vi "InverseMpemba_HotColdWarm.vi"(6 "RN":sgl, 8 "X0":sgl=0.5, 11 "Ring":i16(ring) items=["Cold", "Warm", "Hot"]) -> (3 "Xpot":sgl)   [LabVIEW 2019]
uses:
  <vilib>/Platform/TimedLoop/XDataNode/timing_clust.ctl
  <vilib>/Platform/TimedLoop/XDataNode/nitl_modes.ctl
  <vilib>/Platform/TimedLoop/XDataNode/wakeup.ctl
  <vilib>/rvi/Emulation/niFpgaGetClockAttributes.vi
  <vilib>/rvi/Emulation/niFpgaSctlEmulationGetInTimedLoop.vi
  <vilib>/rvi/Emulation/niFpgaEmulationReportErrorSimple.vi
  <vilib>/rvi/Emulation/niFpgaCriticalErrorInLSC.vi
  <vilib>/Platform/TimedLoop/XDataNode/XDataNode.xnode
  <vilib>/Platform/TimedLoop/XDataNode/XDNodeRunTimeDep.lvlib
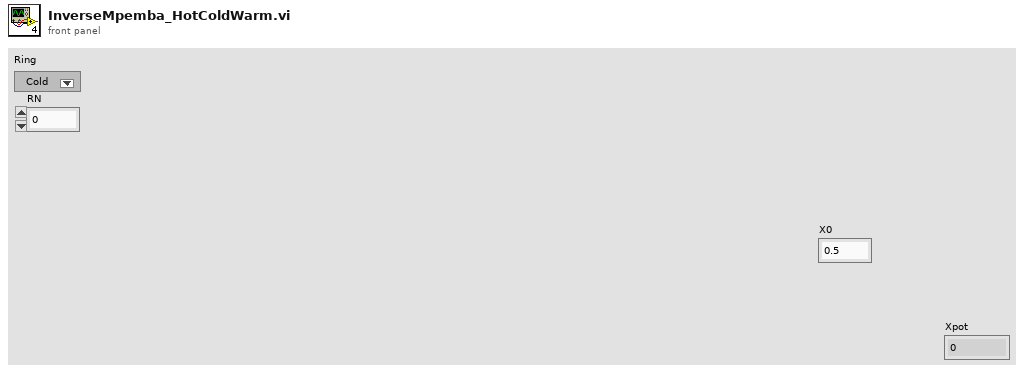
[diagram p1: front panel]
types:
  T1 = typedef "XDNodeRunTimeDep.lvlib/timing_clust.ctl" = cluster{"Expected End [f-1]":u64, "Actual End [f-1]":u64, "Finished Late? [f-1]":bool, "Expected End [i-1]":u64, "Actual End [i-1]":u64, "Finished Late? [i-1]":bool, "Expected Start [i]":u64, "Actual Start [i]":u64, "Expected Start [f]":u64, "Actual Start [f]":u64, "Source Name":string, "Structure Name":string, "Period":i64, "Deadline":i64, "Offset":i64, "Start":i64, "Priority":i32, "Timeout":i32, "Mode":T2, "Wakeup Reason":T3, "Error":errorcluster, "Source Type":string, "Secondary Source Type":string, "Global End Time":u64, "Global Start Time":u64, "Frame Duration":u64, "Iteration Duration":u64, "Assigned CPU":i32, "I/O Scan Engine Mode":u32}
  T2 = typedef "XDNodeRunTimeDep.lvlib/nitl_modes.ctl" = enum32{"No Change", "Process missed periods, maintain original phase", "Discard missed periods, maintain original phase", "Process missed periods, ignore original phase", "Discard missed periods, ignore original phase"}
  T3 = typedef "XDNodeRunTimeDep.lvlib/wakeup.ctl" = enum32{"Normal", "Aborted", "Asynchronous wakeup", "Timing source error", "Timed loop error", "Timeout"}
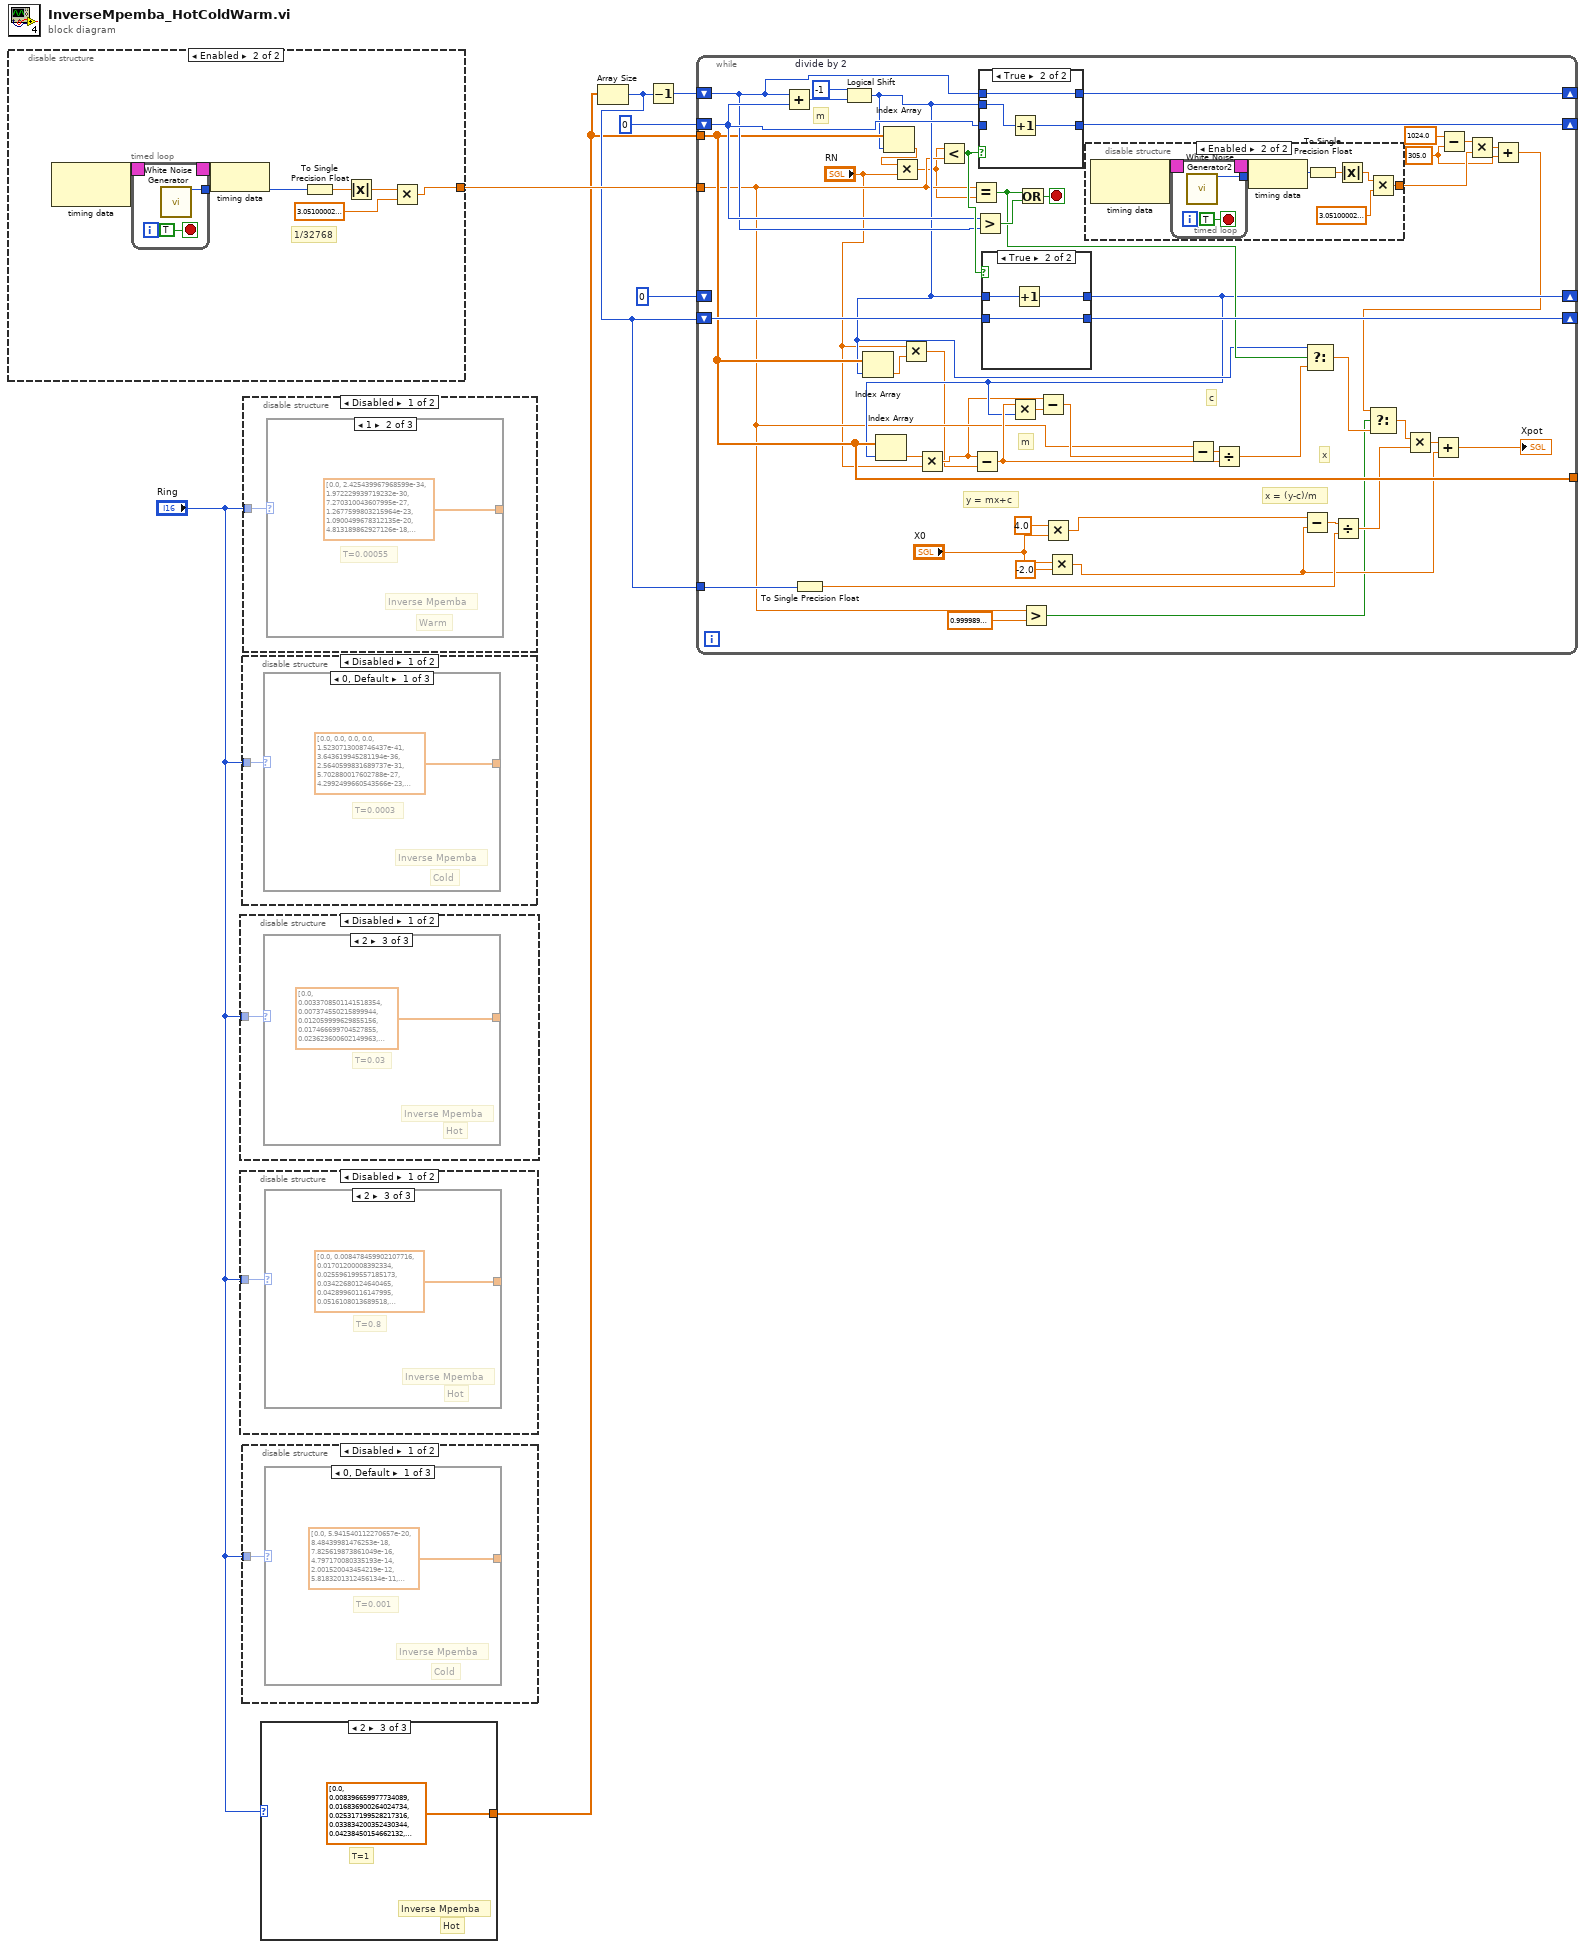
[diagram p0: block diagram]
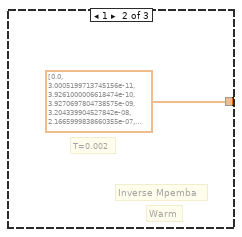
[diagram p2: hidden frame]
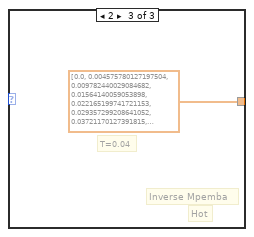
[diagram p3: hidden frame]
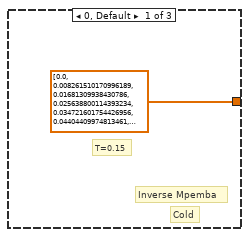
[diagram p5: hidden frame]
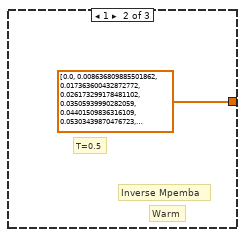
[diagram p6: hidden frame]
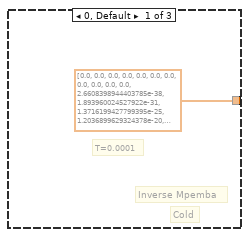
[diagram p7: hidden frame]
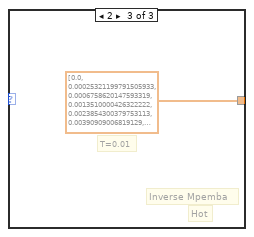
[diagram p8: hidden frame]
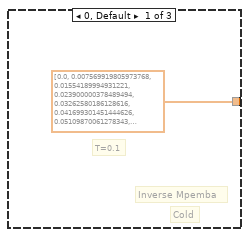
[diagram p10: hidden frame]
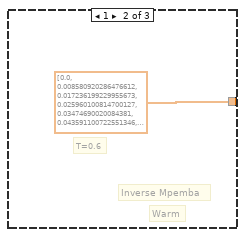
[diagram p11: hidden frame]
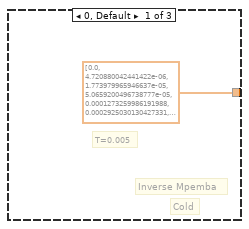
[diagram p13: hidden frame]
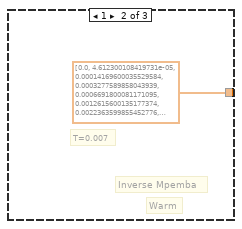
[diagram p14: hidden frame]
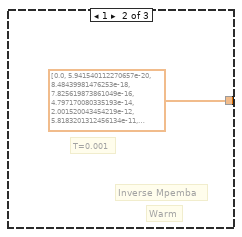
[diagram p16: hidden frame]
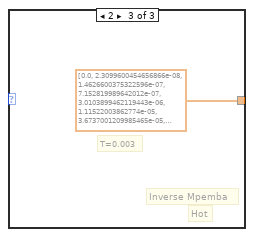
[diagram p17: hidden frame]
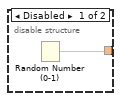
[diagram p19: hidden frame]
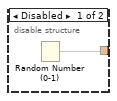
[diagram p20: hidden frame]
diagram:
  n1 = disable-structure shown="Enabled" {
    disable-tunnel: [w8 w11] -> w4
    frame Disabled {
      n2 = Random Number (0-1)() -> (number: 0 to 1=w8:dbl)
    }
    frame Enabled {
      # "1/32768"
      n3 = node-c288() -> (w10:T1)  [unwired: 1 in]
      n4 = timed-loop {
        timing: w10 -> [_]
        timing-out: [_] -> w9
        tunnel: [w17] -> w15
        stop <- TRUE stop-if-true
        n5 = call "White Noise Generator"() -> ("white noise out"=w17:i16)  [unwired: 15 in]
      }
      n6 = node-c288(w9) -> ()
      n7 = To Single Precision Float(number=w15) -> (single precision float=w13:sgl)
      n8 = Absolute Value(x=w13) -> (abs(x)=w12:sgl)
      n9 = Multiply(x=w12, y=sgl 3.051e-05) -> (x*y=w11:sgl)
    }
  }
  n10 = disable-structure shown="Disabled" {
    disable-tunnel: "Ring" -> [w22 _]
    frame Disabled {
      n11 = case shown="2" w22 {
        tunnel: [sgl[] [0.0, 4.72088e-06, 1.77398e-05, 5.06592e-05, 0.000127326, 0.000292503, 0.000623122, 0.0012405, 0.0023204, 0.00409678, 0.00685531, 0.0109145, 0.016595, 0.024182, 0.0338863, 0.0458131, 0.0599432, 0.0761305, 0.0941165, 0.113555, 0.134049, 0.15518, 0.176546, 0.197782, 0.218581, 0.238699, 0.257958, 0.276241, 0.293487, 0.309682, 0.324844, 0.339022, 0.352281, 0.364701, 0.376365, 0.387364, 0.397785, 0.407716, 0.417243, 0.426449, 0.435413, 0.444214, 0.452928, 0.461633, 0.470404, 0.47932, 0.488461, 0.497912, 0.50776, 0.518098, 0.529026, 0.540646, 0.553068, 0.566402, 0.580761, 0.596254, 0.612981, 0.631025, 0.650444, 0.67126, 0.693445, 0.716907, 0.741482, 0.766922, 0.79289, 0.81897, 0.844674, 0.869473, 0.892834, 0.914258, 0.933335, 0.949775, 0.963448, 0.974386, 0.982774, 0.988922, 0.993211, 0.996051, 0.997828, 0.998875, 0.999453, 0.999752, 0.999895, 0.999959, 0.999985, 0.999995, 0.999999, 1.0, 1.0, 1.0, 1.0, 1.0, 1.0, 1.0, 1.0, 1.0, 1.0, 1.0, 1.0, 1.0, 1.0, 1.0, 1.0, 1.0, 1.0, 1.0, 1.0, 1.0, 1.0, 1.0, 1.0, 1.0, 1.0, 1.0, 1.0, 1.0, 1.0, 1.0, 1.0, 1.0, 1.0, 1.0, 1.0, 1.0, 1.0, 1.0, 1.0, 1.0] ("Init Data Out") sgl[] [0.0, 4.6123e-05, 0.000141696, 0.000327759, 0.00066918, 0.00126156, 0.00223636, 0.00376235, 0.0060415, 0.00929849, 0.0137642, 0.0196549, 0.02715, 0.0363724, 0.0473733, 0.0601252, 0.074523, 0.0903924, 0.107505, 0.125596, 0.144383, 0.163587, 0.182944, 0.202216, 0.221204, 0.239745, 0.257717, 0.275033, 0.291642, 0.30752, 0.322669, 0.337109, 0.350874, 0.36401, 0.376572, 0.388616, 0.400206, 0.411404, 0.422275, 0.432883, 0.443291, 0.453564, 0.463765, 0.473957, 0.484205, 0.494573, 0.505128, 0.515936, 0.527067, 0.538591, 0.550581, 0.563108, 0.576246, 0.590066, 0.604637, 0.62002, 0.636269, 0.653422, 0.671499, 0.690496, 0.710378, 0.731071, 0.752462, 0.774387, 0.796638, 0.818956, 0.841044, 0.862574, 0.883202, 0.902591, 0.920434, 0.936475, 0.950531, 0.962511, 0.972417, 0.980344, 0.986469, 0.991025, 0.99428, 0.996507, 0.997962, 0.998868, 0.999403, 0.999702, 0.999859, 0.999938, 0.999974, 0.99999, 0.999996, 0.999999, 1.0, 1.0, 1.0, 1.0, 1.0, 1.0, 1.0, 1.0, 1.0, 1.0, 1.0, 1.0, 1.0, 1.0, 1.0, 1.0, 1.0, 1.0, 1.0, 1.0, 1.0, 1.0, 1.0, 1.0, 1.0, 1.0, 1.0, 1.0, 1.0, 1.0, 1.0, 1.0, 1.0, 1.0, 1.0, 1.0, 1.0, 1.0] ("Init Data Out") sgl[] [0.0, 0.00337085, 0.00737455, 0.01206, 0.0174667, 0.0236236, 0.0305473, 0.0382417, 0.0466981, 0.0558954, 0.0658014, 0.0763735, 0.0875612, 0.0993071, 0.111549, 0.124223, 0.137263, 0.150603, 0.164182, 0.177938, 0.191817, 0.205767, 0.219742, 0.233704, 0.247617, 0.261453, 0.275188, 0.288805, 0.30229, 0.315634, 0.328832, 0.341883, 0.35479, 0.367556, 0.38019, 0.392701, 0.4051, 0.4174, 0.429616, 0.441761, 0.453853, 0.465909, 0.477944, 0.489977, 0.502026, 0.514107, 0.526239, 0.538437, 0.55072, 0.563103, 0.5756, 0.588226, 0.600993, 0.613911, 0.62699, 0.640235, 0.653651, 0.667237, 0.680991, 0.694905, 0.708968, 0.723163, 0.737468, 0.751856, 0.766294, 0.780741, 0.795154, 0.809481, 0.823665, 0.837645, 0.851355, 0.864727, 0.877691, 0.890178, 0.90212, 0.913453, 0.924119, 0.934069, 0.943262, 0.951669, 0.959275, 0.966076, 0.972084, 0.977322, 0.981826, 0.985643, 0.988829, 0.991445, 0.993557, 0.995233, 0.996537, 0.997532, 0.998277, 0.998822, 0.999212, 0.999485, 0.999672, 0.999796, 0.999876, 0.999927, 0.999958, 0.999977, 0.999987, 0.999993, 0.999997, 0.999998, 0.999999, 1.0, 1.0, 1.0, 1.0, 1.0, 1.0, 1.0, 1.0, 1.0, 1.0, 1.0, 1.0, 1.0, 1.0, 1.0, 1.0, 1.0, 1.0, 1.0, 1.0, 1.0] ("Init Data Out")] -> _
        frame 0, Default {
          # "T=0.005"
          # "Inverse Mpemba"
          # "Cold"
        }
        frame 1 {
          # "T=0.007"
          # "Inverse Mpemba"
          # "Warm"
        }
        frame 2 {
          # "T=0.03"
          # "Inverse Mpemba"
          # "Hot"
        }
      }
    }
    frame Enabled {
    }
  }
  n12 = disable-structure shown="Disabled" {
    disable-tunnel: "Ring" -> [w26 _]
    frame Disabled {
      n13 = case shown="2" w26 {
        tunnel: [sgl[] [0.0, 0.00756992, 0.0155419, 0.0239, 0.0326258, 0.0416993, 0.0510987, 0.060801, 0.0707827, 0.0810196, 0.0914873, 0.102162, 0.113019, 0.124037, 0.135192, 0.146464, 0.157833, 0.16928, 0.180787, 0.19234, 0.203924, 0.215525, 0.227133, 0.238737, 0.25033, 0.261903, 0.27345, 0.284968, 0.296452, 0.307899, 0.31931, 0.330682, 0.342016, 0.353313, 0.364574, 0.375803, 0.387001, 0.398173, 0.409321, 0.42045, 0.431565, 0.442669, 0.453768, 0.464866, 0.475968, 0.48708, 0.498205, 0.509349, 0.520516, 0.53171, 0.542935, 0.554194, 0.565491, 0.576828, 0.588207, 0.59963, 0.611096, 0.622606, 0.634158, 0.64575, 0.65738, 0.669042, 0.680731, 0.692441, 0.704162, 0.715887, 0.727602, 0.739297, 0.750956, 0.762565, 0.774106, 0.785561, 0.79691, 0.808131, 0.819203, 0.830103, 0.840806, 0.851287, 0.861522, 0.871486, 0.881155, 0.890504, 0.89951, 0.908153, 0.916412, 0.92427, 0.931712, 0.938726, 0.945303, 0.951436, 0.957124, 0.962368, 0.967173, 0.971547, 0.975503, 0.979054, 0.98222, 0.98502, 0.987478, 0.989617, 0.991463, 0.993042, 0.99438, 0.995504, 0.996437, 0.997206, 0.997831, 0.998334, 0.998735, 0.999051, 0.999296, 0.999484, 0.999627, 0.999734, 0.999813, 0.99987, 0.999911, 0.99994, 0.99996, 0.999974, 0.999984, 0.99999, 0.999994, 0.999996, 0.999998, 0.999999, 1.0, 1.0] ("Init Data Out") sgl[] [0.0, 0.00858092, 0.0172362, 0.0259601, 0.0347469, 0.0435911, 0.0524875, 0.0614311, 0.0704172, 0.0794412, 0.0884988, 0.097586, 0.106699, 0.115834, 0.124988, 0.134158, 0.143342, 0.152535, 0.161737, 0.170945, 0.180157, 0.189371, 0.198586, 0.207801, 0.217014, 0.226224, 0.235431, 0.244634, 0.253833, 0.263027, 0.272215, 0.281399, 0.290578, 0.299751, 0.30892, 0.318084, 0.327244, 0.3364, 0.345554, 0.354704, 0.363853, 0.373, 0.382147, 0.391293, 0.40044, 0.409588, 0.418738, 0.427891, 0.437047, 0.446206, 0.45537, 0.464538, 0.473712, 0.482891, 0.492075, 0.501266, 0.510462, 0.519664, 0.528872, 0.538085, 0.547303, 0.556525, 0.565751, 0.574979, 0.584209, 0.59344, 0.602669, 0.611895, 0.621117, 0.630333, 0.639539, 0.648734, 0.657914, 0.667077, 0.67622, 0.685339, 0.69443, 0.70349, 0.712513, 0.721497, 0.730435, 0.739323, 0.748157, 0.756929, 0.765636, 0.774271, 0.782827, 0.7913, 0.799681, 0.807966, 0.816148, 0.824219, 0.832173, 0.840003, 0.847703, 0.855266, 0.862685, 0.869954, 0.877066, 0.884015, 0.890795, 0.8974, 0.903826, 0.910066, 0.916117, 0.921974, 0.927632, 0.93309, 0.938344, 0.943391, 0.948231, 0.952861, 0.957282, 0.961494, 0.965497, 0.969293, 0.972884, 0.976272, 0.979461, 0.982455, 0.985258, 0.987875, 0.990311, 0.992573, 0.994665, 0.996596, 0.998372, 1.0] ("Init Data Out") sgl[] [0.0, 0.00847846, 0.017012, 0.0255962, 0.0342268, 0.0428996, 0.0516108, 0.0603567, 0.0691336, 0.0779384, 0.0867677, 0.0956186, 0.104488, 0.113374, 0.122274, 0.131186, 0.140107, 0.149035, 0.15797, 0.166909, 0.175851, 0.184794, 0.193738, 0.202682, 0.211625, 0.220566, 0.229504, 0.23844, 0.247372, 0.256301, 0.265226, 0.274147, 0.283064, 0.291978, 0.300889, 0.309796, 0.3187, 0.327602, 0.336501, 0.345398, 0.354294, 0.363189, 0.372083, 0.380977, 0.389871, 0.398767, 0.407664, 0.416563, 0.425464, 0.434367, 0.443274, 0.452184, 0.461098, 0.470016, 0.478938, 0.487864, 0.496795, 0.505729, 0.514668, 0.523611, 0.532557, 0.541507, 0.550459, 0.559413, 0.568368, 0.577323, 0.586278, 0.59523, 0.604179, 0.613124, 0.622062, 0.630991, 0.63991, 0.648816, 0.657708, 0.666582, 0.675436, 0.684267, 0.693071, 0.701846, 0.710588, 0.719293, 0.727958, 0.736578, 0.74515, 0.753668, 0.762128, 0.770526, 0.778857, 0.787115, 0.795295, 0.803393, 0.811403, 0.819319, 0.827136, 0.834848, 0.84245, 0.849936, 0.8573, 0.864538, 0.871644, 0.878611, 0.885436, 0.892113, 0.898637, 0.905003, 0.911208, 0.917246, 0.923114, 0.928808, 0.934326, 0.939664, 0.94482, 0.949791, 0.954577, 0.959175, 0.963586, 0.967809, 0.971845, 0.975693, 0.979356, 0.982835, 0.986133, 0.989251, 0.992193, 0.994962, 0.997563, 1.0] ("Init Data Out")] -> _
        frame 0, Default {
          # "T=0.1"
          # "Inverse Mpemba"
          # "Cold"
        }
        frame 1 {
          # "T=0.6"
          # "Inverse Mpemba"
          # "Warm"
        }
        frame 2 {
          # "T=0.8"
          # "Inverse Mpemba"
          # "Hot"
        }
      }
    }
    frame Enabled {
    }
  }
  n14 = disable-structure shown="Disabled" {
    disable-tunnel: "Ring" -> [w30 _]
    frame Disabled {
      n15 = case shown="0, Default" w30 {
        tunnel: [sgl[] [0.0, 0.0, 0.0, 0.0, 1.52307e-41, 3.64362e-36, 2.56406e-31, 5.70288e-27, 4.29925e-23, 1.17597e-19, 1.2472e-16, 5.4725e-14, 1.05882e-11, 9.62107e-10, 4.37214e-08, 1.05841e-06, 1.45426e-05, 0.000120786, 0.000644813, 0.00234578, 0.00614557, 0.0122228, 0.0194327, 0.025991, 0.0307127, 0.0334893, 0.034865, 0.0354572, 0.0356854, 0.0357664, 0.0357937, 0.0358026, 0.0358055, 0.0358065, 0.0358068, 0.035807, 0.035807, 0.035807, 0.0358071, 0.0358071, 0.0358071, 0.0358071, 0.0358071, 0.0358071, 0.0358071, 0.0358071, 0.0358071, 0.0358071, 0.0358071, 0.0358072, 0.0358073, 0.0358076, 0.0358086, 0.0358119, 0.0358233, 0.0358639, 0.0360097, 0.0365221, 0.0382423, 0.0436096, 0.0587325, 0.0960808, 0.174483, 0.310085, 0.49734, 0.69738, 0.857477, 0.950293, 0.987861, 0.998043, 0.999804, 0.999989, 1.0, 1.0, 1.0, 1.0, 1.0, 1.0, 1.0, 1.0, 1.0, 1.0, 1.0, 1.0, 1.0, 1.0, 1.0, 1.0, 1.0, 1.0, 1.0, 1.0, 1.0, 1.0, 1.0, 1.0, 1.0, 1.0, 1.0, 1.0, 1.0, 1.0, 1.0, 1.0, 1.0, 1.0, 1.0, 1.0, 1.0, 1.0, 1.0, 1.0, 1.0, 1.0, 1.0, 1.0, 1.0, 1.0, 1.0, 1.0, 1.0, 1.0, 1.0, 1.0, 1.0, 1.0, 1.0, 1.0] ("Init Data Out") sgl[] [0.0, 5.94154e-20, 8.4844e-18, 7.82562e-16, 4.79717e-14, 2.00152e-12, 5.81832e-11, 1.20575e-09, 1.82176e-08, 2.05116e-07, 1.75793e-06, 1.17058e-05, 6.1769e-05, 0.000263223, 0.000922445, 0.00270504, 0.00674966, 0.0145632, 0.0275964, 0.0466214, 0.0712428, 0.0998487, 0.130049, 0.159361, 0.185814, 0.208252, 0.226325, 0.240289, 0.250735, 0.258369, 0.263866, 0.267796, 0.270606, 0.272631, 0.27411, 0.27521, 0.276049, 0.276708, 0.277242, 0.277691, 0.278084, 0.278443, 0.278784, 0.279123, 0.279475, 0.279857, 0.280291, 0.280804, 0.281436, 0.282242, 0.283308, 0.28476, 0.28679, 0.289687, 0.293886, 0.300029, 0.30904, 0.322196, 0.34117, 0.367978, 0.404757, 0.453305, 0.514361, 0.586776, 0.666913, 0.748743, 0.82496, 0.888943, 0.936757, 0.96816, 0.986048, 0.994764, 0.998345, 0.999567, 0.999908, 0.999984, 0.999998, 1.0, 1.0, 1.0, 1.0, 1.0, 1.0, 1.0, 1.0, 1.0, 1.0, 1.0, 1.0, 1.0, 1.0, 1.0, 1.0, 1.0, 1.0, 1.0, 1.0, 1.0, 1.0, 1.0, 1.0, 1.0, 1.0, 1.0, 1.0, 1.0, 1.0, 1.0, 1.0, 1.0, 1.0, 1.0, 1.0, 1.0, 1.0, 1.0, 1.0, 1.0, 1.0, 1.0, 1.0, 1.0, 1.0, 1.0, 1.0, 1.0, 1.0, 1.0] ("Init Data Out") sgl[] [0.0, 2.30996e-08, 1.46266e-07, 7.15282e-07, 3.01039e-06, 1.11522e-05, 3.6737e-05, 0.000108448, 0.000288933, 0.000699502, 0.00154899, 0.00315746, 0.00596125, 0.0104867, 0.0172879, 0.0268576, 0.0395304, 0.055406, 0.0743127, 0.0958207, 0.1193, 0.144005, 0.169167, 0.194078, 0.218141, 0.240907, 0.262077, 0.281493, 0.299111, 0.314975, 0.329191, 0.341902, 0.353271, 0.363464, 0.372645, 0.380968, 0.388576, 0.395596, 0.402146, 0.408332, 0.414249, 0.419987, 0.425632, 0.431265, 0.436971, 0.442835, 0.448949, 0.455411, 0.462334, 0.469841, 0.478075, 0.487199, 0.497396, 0.508873, 0.521858, 0.536597, 0.553344, 0.572345, 0.59382, 0.617927, 0.644731, 0.674153, 0.705933, 0.739594, 0.774426, 0.809506, 0.84375, 0.876018, 0.905238, 0.930553, 0.951434, 0.967756, 0.979783, 0.988095, 0.993454, 0.996658, 0.998426, 0.99932, 0.999733, 0.999905, 0.99997, 0.999991, 0.999998, 1.0, 1.0, 1.0, 1.0, 1.0, 1.0, 1.0, 1.0, 1.0, 1.0, 1.0, 1.0, 1.0, 1.0, 1.0, 1.0, 1.0, 1.0, 1.0, 1.0, 1.0, 1.0, 1.0, 1.0, 1.0, 1.0, 1.0, 1.0, 1.0, 1.0, 1.0, 1.0, 1.0, 1.0, 1.0, 1.0, 1.0, 1.0, 1.0, 1.0, 1.0, 1.0, 1.0, 1.0, 1.0] ("Init Data Out")] -> _
        frame 0, Default {
          # "T=0.0003"
          # "Inverse Mpemba"
          # "Cold"
        }
        frame 1 {
          # "T=0.001"
          # "Inverse Mpemba"
          # "Warm"
        }
        frame 2 {
          # "T=0.003"
          # "Inverse Mpemba"
          # "Hot"
        }
      }
    }
    frame Enabled {
    }
  }
  n16 = disable-structure shown="Disabled" {
    disable-tunnel: "Ring" -> [w34 _]
    frame Disabled {
      n17 = case shown="0, Default" w34 {
        tunnel: [sgl[] [0.0, 5.94154e-20, 8.4844e-18, 7.82562e-16, 4.79717e-14, 2.00152e-12, 5.81832e-11, 1.20575e-09, 1.82176e-08, 2.05116e-07, 1.75793e-06, 1.17058e-05, 6.1769e-05, 0.000263223, 0.000922445, 0.00270504, 0.00674966, 0.0145632, 0.0275964, 0.0466214, 0.0712428, 0.0998487, 0.130049, 0.159361, 0.185814, 0.208252, 0.226325, 0.240289, 0.250735, 0.258369, 0.263866, 0.267796, 0.270606, 0.272631, 0.27411, 0.27521, 0.276049, 0.276708, 0.277242, 0.277691, 0.278084, 0.278443, 0.278784, 0.279123, 0.279475, 0.279857, 0.280291, 0.280804, 0.281436, 0.282242, 0.283308, 0.28476, 0.28679, 0.289687, 0.293886, 0.300029, 0.30904, 0.322196, 0.34117, 0.367978, 0.404757, 0.453305, 0.514361, 0.586776, 0.666913, 0.748743, 0.82496, 0.888943, 0.936757, 0.96816, 0.986048, 0.994764, 0.998345, 0.999567, 0.999908, 0.999984, 0.999998, 1.0, 1.0, 1.0, 1.0, 1.0, 1.0, 1.0, 1.0, 1.0, 1.0, 1.0, 1.0, 1.0, 1.0, 1.0, 1.0, 1.0, 1.0, 1.0, 1.0, 1.0, 1.0, 1.0, 1.0, 1.0, 1.0, 1.0, 1.0, 1.0, 1.0, 1.0, 1.0, 1.0, 1.0, 1.0, 1.0, 1.0, 1.0, 1.0, 1.0, 1.0, 1.0, 1.0, 1.0, 1.0, 1.0, 1.0, 1.0, 1.0, 1.0, 1.0] ("Init Data Out") sgl[] [0.0, 3.00052e-11, 3.9261e-10, 3.92707e-09, 3.20434e-08, 2.1666e-07, 1.22831e-06, 5.90395e-06, 2.43181e-05, 8.6726e-05, 0.000270482, 0.00074488, 0.00182828, 0.0040358, 0.00808229, 0.0148089, 0.0250284, 0.0393249, 0.0578756, 0.0803594, 0.105987, 0.133639, 0.162059, 0.190055, 0.216638, 0.241106, 0.263052, 0.282331, 0.298998, 0.313241, 0.325323, 0.335539, 0.34418, 0.351515, 0.357785, 0.363197, 0.367924, 0.372115, 0.375891, 0.379355, 0.382597, 0.385692, 0.388711, 0.391722, 0.394791, 0.397989, 0.401393, 0.405094, 0.409197, 0.413832, 0.419157, 0.425369, 0.43271, 0.441476, 0.452028, 0.464788, 0.480242, 0.498918, 0.521356, 0.548039, 0.579314, 0.615274, 0.655631, 0.699613, 0.745903, 0.792685, 0.837813, 0.879109, 0.914723, 0.943477, 0.96506, 0.980014, 0.989506, 0.994985, 0.997837, 0.999166, 0.999715, 0.999915, 0.999978, 0.999995, 0.999999, 1.0, 1.0, 1.0, 1.0, 1.0, 1.0, 1.0, 1.0, 1.0, 1.0, 1.0, 1.0, 1.0, 1.0, 1.0, 1.0, 1.0, 1.0, 1.0, 1.0, 1.0, 1.0, 1.0, 1.0, 1.0, 1.0, 1.0, 1.0, 1.0, 1.0, 1.0, 1.0, 1.0, 1.0, 1.0, 1.0, 1.0, 1.0, 1.0, 1.0, 1.0, 1.0, 1.0, 1.0, 1.0, 1.0, 1.0] ("Init Data Out") sgl[] [0.0, 0.00457578, 0.00978244, 0.0156414, 0.0221652, 0.0293573, 0.0372117, 0.0457137, 0.0548401, 0.0645603, 0.0748372, 0.0856285, 0.0968879, 0.108566, 0.120613, 0.132977, 0.145608, 0.158457, 0.171477, 0.184626, 0.197861, 0.211148, 0.224453, 0.237748, 0.251009, 0.264214, 0.277347, 0.290395, 0.303348, 0.3162, 0.328946, 0.341585, 0.354119, 0.366551, 0.378887, 0.391131, 0.403294, 0.415384, 0.427411, 0.439387, 0.451323, 0.463232, 0.475126, 0.487019, 0.498923, 0.510851, 0.522816, 0.534832, 0.546909, 0.559059, 0.571294, 0.583623, 0.596056, 0.608599, 0.621258, 0.634038, 0.646941, 0.659967, 0.673114, 0.686375, 0.699742, 0.713203, 0.726743, 0.740342, 0.753975, 0.767616, 0.781232, 0.794787, 0.808241, 0.821549, 0.834663, 0.847535, 0.860111, 0.872338, 0.884162, 0.895531, 0.906394, 0.916705, 0.926421, 0.935508, 0.943936, 0.951686, 0.958746, 0.965116, 0.970804, 0.975827, 0.980213, 0.983996, 0.987217, 0.989924, 0.992167, 0.993998, 0.995471, 0.996636, 0.997542, 0.998235, 0.998755, 0.999139, 0.999415, 0.999611, 0.999747, 0.999839, 0.9999, 0.999939, 0.999964, 0.999979, 0.999988, 0.999994, 0.999997, 0.999998, 0.999999, 1.0, 1.0, 1.0, 1.0, 1.0, 1.0, 1.0, 1.0, 1.0, 1.0, 1.0, 1.0, 1.0, 1.0, 1.0, 1.0, 1.0] ("Init Data Out")] -> _
        frame 0, Default {
          # "T=0.001"
          # "Inverse Mpemba"
          # "Cold"
        }
        frame 1 {
          # "T=0.002"
          # "Inverse Mpemba"
          # "Warm"
        }
        frame 2 {
          # "T=0.04"
          # "Inverse Mpemba"
          # "Hot"
        }
      }
    }
    frame Enabled {
    }
  }
  n18 = disable-structure shown="Disabled" {
    disable-tunnel: "Ring" -> [w38 _]
    frame Disabled {
      n19 = case shown="1" w38 {
        tunnel: [sgl[] [0.0, 0.0, 0.0, 0.0, 0.0, 0.0, 0.0, 0.0, 0.0, 0.0, 0.0, 2.66084e-38, 1.89396e-31, 1.37162e-25, 1.20369e-20, 1.51581e-16, 3.22645e-13, 1.36189e-10, 1.33848e-08, 3.64184e-07, 3.36451e-06, 1.33789e-05, 2.88128e-05, 4.0894e-05, 4.58943e-05, 4.7037e-05, 4.71912e-05, 4.72046e-05, 4.72054e-05, 4.72055e-05, 4.72055e-05, 4.72055e-05, 4.72055e-05, 4.72055e-05, 4.72055e-05, 4.72055e-05, 4.72055e-05, 4.72055e-05, 4.72055e-05, 4.72055e-05, 4.72055e-05, 4.72055e-05, 4.72055e-05, 4.72055e-05, 4.72055e-05, 4.72055e-05, 4.72055e-05, 4.72055e-05, 4.72055e-05, 4.72055e-05, 4.72055e-05, 4.72055e-05, 4.72055e-05, 4.72055e-05, 4.72055e-05, 4.72055e-05, 4.72057e-05, 4.72164e-05, 4.76069e-05, 5.88841e-05, 0.000293518, 0.00350145, 0.0298047, 0.148844, 0.428559, 0.75934, 0.948955, 0.995786, 0.999894, 0.999999, 1.0, 1.0, 1.0, 1.0, 1.0, 1.0, 1.0, 1.0, 1.0, 1.0, 1.0, 1.0, 1.0, 1.0, 1.0, 1.0, 1.0, 1.0, 1.0, 1.0, 1.0, 1.0, 1.0, 1.0, 1.0, 1.0, 1.0, 1.0, 1.0, 1.0, 1.0, 1.0, 1.0, 1.0, 1.0, 1.0, 1.0, 1.0, 1.0, 1.0, 1.0, 1.0, 1.0, 1.0, 1.0, 1.0, 1.0, 1.0, 1.0, 1.0, 1.0, 1.0, 1.0, 1.0, 1.0, 1.0, 1.0, 1.0] ("Init Data Out") sgl[] [0.0, 2.42544e-34, 1.97223e-30, 7.27031e-27, 1.26776e-23, 1.09005e-20, 4.81319e-18, 1.13584e-15, 1.48979e-13, 1.12882e-11, 5.13322e-10, 1.45473e-08, 2.66648e-07, 3.27867e-06, 2.80206e-05, 0.000172244, 0.000786891, 0.00275621, 0.00762456, 0.017138, 0.0321714, 0.0518015, 0.0734251, 0.0939255, 0.11098, 0.123667, 0.132261, 0.137656, 0.140848, 0.142656, 0.143652, 0.144194, 0.144488, 0.14465, 0.144741, 0.144794, 0.144827, 0.144847, 0.144862, 0.144872, 0.14488, 0.144887, 0.144893, 0.144899, 0.144906, 0.144914, 0.144923, 0.144936, 0.144956, 0.144986, 0.145036, 0.145125, 0.145288, 0.1456, 0.146213, 0.14744, 0.149903, 0.154798, 0.164305, 0.182074, 0.213533, 0.265424, 0.343793, 0.450232, 0.577832, 0.710283, 0.826998, 0.912547, 0.963611, 0.98789, 0.996871, 0.999391, 0.999914, 0.999991, 0.999999, 1.0, 1.0, 1.0, 1.0, 1.0, 1.0, 1.0, 1.0, 1.0, 1.0, 1.0, 1.0, 1.0, 1.0, 1.0, 1.0, 1.0, 1.0, 1.0, 1.0, 1.0, 1.0, 1.0, 1.0, 1.0, 1.0, 1.0, 1.0, 1.0, 1.0, 1.0, 1.0, 1.0, 1.0, 1.0, 1.0, 1.0, 1.0, 1.0, 1.0, 1.0, 1.0, 1.0, 1.0, 1.0, 1.0, 1.0, 1.0, 1.0, 1.0, 1.0, 1.0, 1.0] ("Init Data Out") sgl[] [0.0, 0.000253212, 0.000675862, 0.001351, 0.00238543, 0.00390909, 0.00607125, 0.00903351, 0.0129599, 0.0180051, 0.0243018, 0.0319498, 0.0410065, 0.0514818, 0.0633368, 0.0764859, 0.0908035, 0.106132, 0.122293, 0.139097, 0.156351, 0.173873, 0.191492, 0.209057, 0.22644, 0.243536, 0.260262, 0.276559, 0.292386, 0.307723, 0.322564, 0.336914, 0.350792, 0.364223, 0.37724, 0.389879, 0.402183, 0.414195, 0.425959, 0.437524, 0.448936, 0.460244, 0.471496, 0.482742, 0.49403, 0.505412, 0.516936, 0.528653, 0.540614, 0.552869, 0.565468, 0.57846, 0.591892, 0.605808, 0.62025, 0.63525, 0.650836, 0.667025, 0.683819, 0.701207, 0.719158, 0.73762, 0.756515, 0.77574, 0.795164, 0.814629, 0.833954, 0.852934, 0.871354, 0.888992, 0.90563, 0.921072, 0.935148, 0.947731, 0.958742, 0.968159, 0.976016, 0.9824, 0.987441, 0.991303, 0.994166, 0.996218, 0.997636, 0.998577, 0.999178, 0.999545, 0.99976, 0.999879, 0.999942, 0.999974, 0.999989, 0.999995, 0.999998, 0.999999, 1.0, 1.0, 1.0, 1.0, 1.0, 1.0, 1.0, 1.0, 1.0, 1.0, 1.0, 1.0, 1.0, 1.0, 1.0, 1.0, 1.0, 1.0, 1.0, 1.0, 1.0, 1.0, 1.0, 1.0, 1.0, 1.0, 1.0, 1.0, 1.0, 1.0, 1.0, 1.0, 1.0, 1.0] ("Init Data Out")] -> _
        frame 0, Default {
          # "T=0.0001"
          # "Inverse Mpemba"
          # "Cold"
        }
        frame 1 {
          # "T=0.00055"
          # "Inverse Mpemba"
          # "Warm"
        }
        frame 2 {
          # "T=0.01"
          # "Inverse Mpemba"
          # "Hot"
        }
      }
    }
    frame Enabled {
    }
  }
  n20 = case shown="2" "Ring" {
    tunnel: [sgl[] [0.0, 0.00826151, 0.0168131, 0.0256388, 0.0347216, 0.0440441, 0.0535885, 0.0633371, 0.073272, 0.0833755, 0.0936303, 0.10402, 0.114528, 0.125139, 0.135838, 0.146612, 0.157447, 0.168332, 0.179255, 0.190207, 0.201179, 0.212161, 0.223148, 0.234133, 0.245109, 0.256074, 0.267023, 0.277952, 0.288861, 0.299746, 0.310608, 0.321445, 0.332259, 0.343048, 0.353815, 0.364561, 0.375288, 0.385998, 0.396693, 0.407375, 0.418048, 0.428715, 0.439378, 0.450041, 0.460707, 0.471378, 0.482058, 0.49275, 0.503456, 0.51418, 0.524924, 0.53569, 0.54648, 0.557295, 0.568137, 0.579006, 0.589903, 0.600828, 0.61178, 0.622757, 0.633757, 0.644778, 0.655816, 0.666867, 0.677925, 0.688985, 0.70004, 0.711081, 0.7221, 0.733088, 0.744032, 0.754922, 0.765745, 0.776486, 0.787132, 0.797667, 0.808075, 0.818339, 0.828441, 0.838364, 0.84809, 0.8576, 0.866877, 0.875902, 0.884658, 0.893128, 0.901296, 0.909147, 0.916669, 0.923849, 0.930676, 0.937144, 0.943245, 0.948975, 0.954333, 0.95932, 0.963939, 0.968195, 0.972095, 0.975651, 0.978874, 0.981778, 0.984379, 0.986692, 0.988738, 0.990533, 0.992098, 0.993453, 0.994616, 0.995607, 0.996445, 0.997148, 0.997732, 0.998213, 0.998606, 0.998924, 0.999178, 0.99938, 0.999539, 0.999662, 0.999757, 0.999829, 0.999883, 0.999923, 0.999952, 0.999974, 0.999989, 1.0] ("Init Data Out") sgl[] [0.0, 0.00863681, 0.0173636, 0.0261733, 0.0350594, 0.0440151, 0.0530344, 0.0621111, 0.0712395, 0.0804142, 0.0896298, 0.0988817, 0.108165, 0.117476, 0.126809, 0.136162, 0.145532, 0.154914, 0.164306, 0.173705, 0.183109, 0.192517, 0.201925, 0.211333, 0.220739, 0.230141, 0.23954, 0.248933, 0.258321, 0.267704, 0.27708, 0.286449, 0.295813, 0.30517, 0.314522, 0.323868, 0.333209, 0.342545, 0.351878, 0.361207, 0.370534, 0.379859, 0.389184, 0.398508, 0.407833, 0.417159, 0.426488, 0.43582, 0.445155, 0.454496, 0.463841, 0.473192, 0.482549, 0.491913, 0.501284, 0.510662, 0.520048, 0.52944, 0.538839, 0.548245, 0.557657, 0.567074, 0.576495, 0.58592, 0.595347, 0.604774, 0.6142, 0.623622, 0.633038, 0.642447, 0.651844, 0.661228, 0.670594, 0.679938, 0.689258, 0.698549, 0.707805, 0.717023, 0.726198, 0.735323, 0.744393, 0.753403, 0.762345, 0.771214, 0.780003, 0.788705, 0.797312, 0.805818, 0.814215, 0.822495, 0.830652, 0.838677, 0.846562, 0.854301, 0.861885, 0.869307, 0.87656, 0.883637, 0.890532, 0.897237, 0.903748, 0.910058, 0.916162, 0.922055, 0.927734, 0.933196, 0.938437, 0.943455, 0.948248, 0.952817, 0.957161, 0.961281, 0.965179, 0.968856, 0.972315, 0.975561, 0.978598, 0.98143, 0.984064, 0.986506, 0.988761, 0.990839, 0.992745, 0.994489, 0.996078, 0.99752, 0.998825, 1.0] ("Init Data Out") sgl[] [0.0, 0.00839666, 0.0168369, 0.0253172, 0.0338342, 0.0423845, 0.0509651, 0.0595729, 0.0682053, 0.0768594, 0.0855329, 0.0942234, 0.102929, 0.111647, 0.120376, 0.129114, 0.137859, 0.146611, 0.155367, 0.164126, 0.172888, 0.181651, 0.190415, 0.199178, 0.207941, 0.216702, 0.225461, 0.234218, 0.242972, 0.251724, 0.260472, 0.269218, 0.277961, 0.286701, 0.295438, 0.304172, 0.312905, 0.321635, 0.330363, 0.33909, 0.347816, 0.356541, 0.365265, 0.37399, 0.382714, 0.39144, 0.400166, 0.408894, 0.417624, 0.426356, 0.435091, 0.443828, 0.452567, 0.46131, 0.470057, 0.478806, 0.487559, 0.496316, 0.505075, 0.513837, 0.522603, 0.531371, 0.54014, 0.548912, 0.557684, 0.566456, 0.575228, 0.583998, 0.592766, 0.60153, 0.610288, 0.61904, 0.627784, 0.636518, 0.645241, 0.653949, 0.662642, 0.671317, 0.679971, 0.688602, 0.697206, 0.705782, 0.714326, 0.722835, 0.731305, 0.739733, 0.748116, 0.756449, 0.764728, 0.772949, 0.781109, 0.789203, 0.797226, 0.805174, 0.813042, 0.820826, 0.82852, 0.836121, 0.843623, 0.851022, 0.858311, 0.865488, 0.872547, 0.879483, 0.886291, 0.892968, 0.899508, 0.905908, 0.912163, 0.91827, 0.924225, 0.930023, 0.935663, 0.941141, 0.946455, 0.951602, 0.95658, 0.961388, 0.966024, 0.970487, 0.974778, 0.978895, 0.982839, 0.98661, 0.990211, 0.993641, 0.996903, 1.0] ("Init Data Out")] -> w1
    frame 0, Default {
      # "T=0.15"
      # "Inverse Mpemba"
      # "Cold"
    }
    frame 1 {
      # "T=0.5"
      # "Inverse Mpemba"
      # "Warm"
    }
    frame 2 {
      # "T=1"
      # "Inverse Mpemba"
      # "Hot"
    }
  }
  n21 = Array Size(array=w1) -> (size(s)=w3:i32)
  n22 = Decrement(x=w3) -> (x-1=w5:i32)
  n23 = while {
    tunnel: w1 -> [w82]
    tunnel: w4 -> [w63]
    shift-right: [w92] -> _
    shift-left: w5 -> [w83]
    shift-right: [w88] -> _
    shift-left: 0 -> [w84]
    shift-right: [w74] -> _
    shift-left: 0 -> [_]
    shift-right: [w85] -> _
    shift-left: w3 -> [w86]
    tunnel: [w82] -> _
    tunnel: w3 -> [w68]
    stop <- w90 stop-if-true
    w56 = sgl 305.0 ("y")
    w93 = -1  # divide by 2
    # "x"
    # "x = (y-c)/m"
    # "c"
    # "m"
    # "y = mx+c"
    # "m"
    n24 = Add(x=w83, y=w84) -> (x+y=w89:i32)
    n25 = To Single Precision Float(number=w68) -> (single precision float=w67:sgl)
    n26 = Logical Shift(y=w93, x=w89) -> (x << y=w80:i32)
    n27 = Index Array(array=w82, index=w80) -> (element=w48:sgl)
    n28 = Index Array(array=w82, index=w80) -> (element=w52:sgl)
    n29 = Multiply(x=w52, y="RN") -> (x*y=w51:sgl)
    n30 = Multiply(x="RN", y=w48) -> (x*y=w46:sgl)
    n31 = Less?(x=w51, y=w63) -> (x < y?=w87:bool)
    n32 = Equal?(x=w63, y=w51) -> (x = y?=w81:bool)
    n33 = Greater?(x=w84, y=w83) -> (0:w91:bool)
    n34 = case shown="True" w87 {
      tunnel: w80 -> [w115 w118]
      tunnel: [w114 w116] -> w92
      tunnel: w84 -> [w113 _]
      tunnel: [w113 w117] -> w88
      tunnel: w83 -> [_ w116]
      frame False {
        n35 = Decrement(x=w115) -> (x-1=w114:i32)
      }
      frame True {
        n36 = Increment(x=w118) -> (x+1=w117:i32)
      }
    }
    n37 = case shown="True" w87 {
      tunnel: w80 -> [w109 w112]
      tunnel: [w108 w111] -> w74
      tunnel: w86 -> [w108 w110]
      tunnel: [w109 w110] -> w85
      frame False {
      }
      frame True {
        n38 = Increment(x=w112) -> (x+1=w111:i32)
      }
    }
    n39 = Index Array(array=w82, index=w74) -> (element=w50:sgl)
    n40 = Multiply(x=w50, y="RN") -> (x*y=w49:sgl)
    n41 = Subtract(x=w49, y=w46) -> (x-y=w76:sgl)
    n42 = Multiply(x=w76, y=w74) -> (x*y=w79:sgl)
    n43 = Or(x=w81, y=w91) -> (x .or. y?=w90:bool)
    n44 = Greater?(x=w63, y=sgl 0.99999) -> (0:w53:bool)
    n45 = Subtract(x=w49, y=w79) -> (x-y=w78:sgl)
    n46 = Multiply(x=sgl 4.0, y="X0") -> (x*y=w71:sgl)
    n47 = Multiply(x="X0", y=sgl -2.0) -> (x*y=w65:sgl)
    n48 = disable-structure shown="Enabled" {
      disable-tunnel: [w94 w97] -> w58
      frame Disabled {
        n49 = Random Number (0-1)() -> (number: 0 to 1=w94:dbl)
      }
      frame Enabled {
        n50 = node-c288() -> (w96:T1)  [unwired: 1 in]
        n51 = timed-loop {
          timing: w96 -> [_]
          timing-out: [_] -> w95
          tunnel: [w103] -> w101
          stop <- TRUE stop-if-true
          n52 = call "White Noise Generator2"() -> ("white noise out"=w103:i16)  [unwired: 15 in]
        }
        n53 = node-c288(w95) -> ()
        n54 = To Single Precision Float(number=w101) -> (single precision float=w99:sgl)
        n55 = Absolute Value(x=w99) -> (abs(x)=w98:sgl)
        n56 = Multiply(x=w98, y=sgl 3.051e-05) -> (x*y=w97:sgl)
      }
    }
    n57 = Subtract(x=w63, y=w78) -> (x-y=w77:sgl)
    n58 = Divide(x=w77, y=w76) -> (x/y=w75:sgl)
    n59 = Subtract(x=w71, y=w65) -> (x-y=w70:sgl)
    n60 = Select(t=w80, s=w81, f=w75) -> (s? t:f=w61:sgl)
    n61 = Divide(x=w70, y=w67) -> (x/y=w69:sgl)
    n62 = Subtract(x=sgl 1024.0, y=w56) -> (x-y=w59:sgl)
    n63 = Multiply(x=w59, y=w58) -> (x*y=w57:sgl)
    n64 = Add(x=w57, y=w56) -> (x+y=w54:sgl)
    n65 = Select(t=w54, s=w53, f=w61) -> (s? t:f=w55:sgl)
    n66 = Multiply(x=w55, y=w69) -> (x*y=w66:sgl)
    n67 = Add(x=w66, y=w65) -> (x+y=→"Xpot":sgl)
  }
